vi "GetKE2510PathStringFromJson.vi"(2 "Error In":errorcluster, 3 "JSON":string) -> (0 "Error Out":errorcluster, 1 "Path String":string)   [LabVIEW 2014]
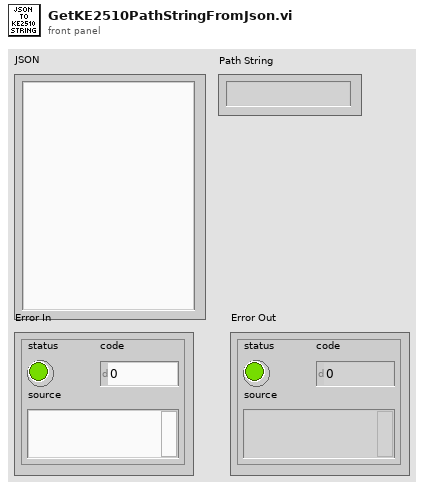
[diagram p1: front panel]
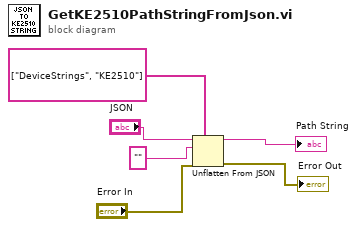
[diagram p0: block diagram]
diagram:
  n1 = Unflatten From JSON(path=string[] ["DeviceStrings", "KE2510"], JSON string="JSON", type and defaults="", error in (no error)="Error In") -> (value=→"Path String":string, error out=→"Error Out":errorcluster)  [unwired: 3 in]
